vi "Write DAQ.vi"(8 "error in (no error)":errorcluster, 10 "DAQ":T1={"AO Fs (Hz)"=100000.0, "DO Fs (Hz)"=25000.0, "Poll Rate (Hz)"=50.0, "Baseline (s)"=50.0}, 11 "Parameters in":refnum<class "Parameters.lvclass">) -> (0 "error out":errorcluster, 3 "Parameters out":refnum<class "Parameters.lvclass">)   [LabVIEW 2020, in "Parameters.lvclass"]
uses:
  Parameters.lvclass
  DAQ.ctl
  Parameters.lvclass/Parameters.ctl
  State/State.lvclass
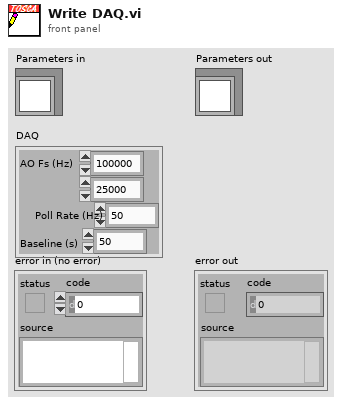
[diagram p1: front panel]
types:
  T1 = typedef "Parameters.lvclass/DAQ.ctl" = cluster{"AO Fs (Hz)":dbl, "DO Fs (Hz)":dbl, "Poll Rate (Hz)":dbl, "Baseline (s)":dbl}
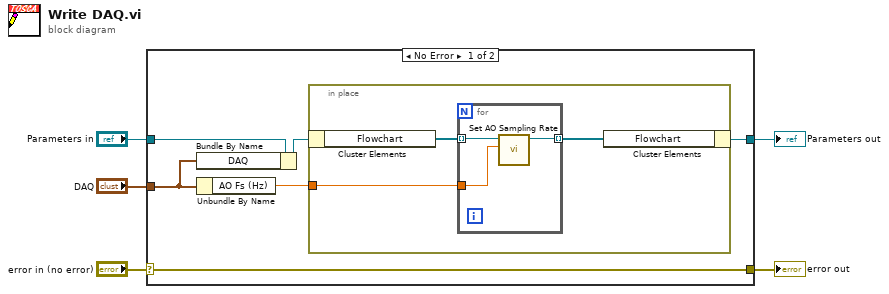
[diagram p0: block diagram]
diagram:
  n1 = case shown="No Error" "error in (no error)" {
    selector: "error in (no error)" -> [w11 w18]
    tunnel: [w11 w18] -> w4
    tunnel: [w7 w19] -> w2
    tunnel: "Parameters in" -> [w10 w19]
    tunnel: "DAQ" -> [w9 _]
    frame No Error {
      n2 = Bundle By Name(cluster=w10, "DAQ"=w9) -> (w8:refnum<class "Parameters.lvclass">)
      n3 = Unbundle By Name(w9) -> ("AO Fs (Hz)"=w6:dbl)
      n4 = in-place {
        in-place-border: w6 -> [w12]
        n5 = in-place-cluster #1(w8) -> ("Flowchart"=w14:refnum<class "State.lvclass">[])
        n6 = for {
          tunnel: w14 -> [w17] mode=indexing
          tunnel: [w15] -> w13 mode=indexing
          tunnel: w12 -> [w16]
          n7 = call "Set AO Sampling Rate.vi"("Fs (Hz)"=w16, "State in"=w17) -> ("State out"=w15:refnum<class "State.lvclass">)  [unwired: 8 in, 1 out]
        }
        n8 = in-place-cluster #1("Flowchart"=w13) -> (w7:refnum<class "Parameters.lvclass">)
      }
    }
    frame Error {
    }
  }
  "error out" <- w4
  "Parameters out" <- w2
